vi "LVClasse_Intensity GetStatisticDatas.vi"(0 "Phase in":refnum<class "Intensity.lvclass">, 11 "error in (no error)":errorcluster) -> (4 "Phase out":refnum<class "Intensity.lvclass">, 6 "StatisticsData":T1, 15 "error out":errorcluster)   [LabVIEW 2020, in "Intensity.lvclass"]
doc: "Phase statistic data getter.\n\n--------------------------------------------------------------------------------\n\n<B>PhaseIn </B> : Phase object.\n<B>PhaseOut </B> : Phase object.\n<B>rms </B> : Phase root mean square deviation.\n<B>pv </B> : Phase peak to valley.\n<B>max </B> : Phase maximum.\n<B>min </B> : Phase minimum.\n<B>ErrorIn </B> : Error\n<B>ErrorOut </B> : Error\n\n--------------------------------------------------------------------------------"
uses:
  Intensity.lvclass
  StatisticsData.ctl
  Intensity.lvclass/Intensity.ctl
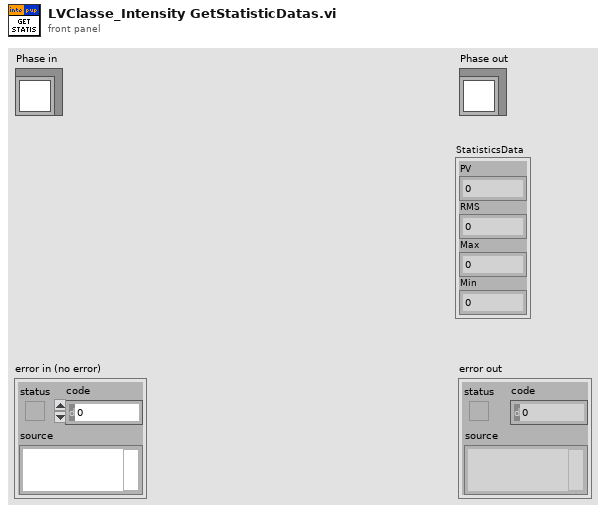
[diagram p1: front panel]
types:
  T1 = typedef "StatisticsData.ctl" = cluster{"PV":sgl, "RMS":dbl, "Max":sgl, "Min":sgl}
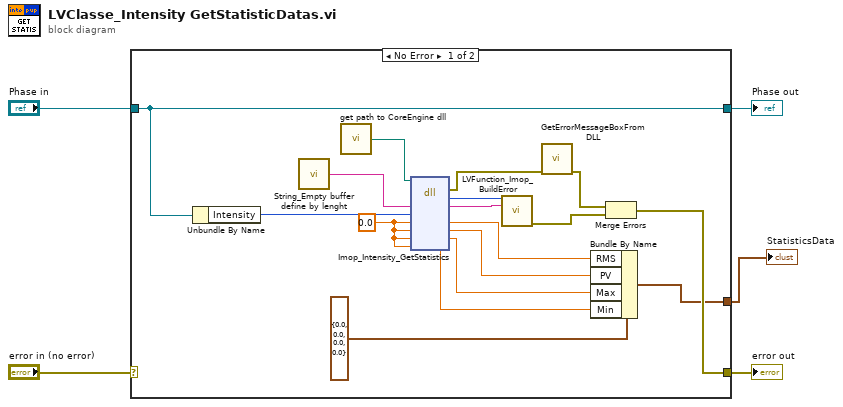
[diagram p0: block diagram]
diagram:
  n1 = case shown="No Error" "error in (no error)" {
    selector: "error in (no error)" -> [_ w24]
    tunnel: [w13 w24] -> w4
    tunnel: [w14 w23] -> w2
    tunnel: "Phase in" -> [w14 w23]
    tunnel: [w12 _] -> w1
    frame No Error {
      w6 = 0.0 ("rms")
      n2 = Unbundle By Name(w14) -> ("Intensity"=w17:i32)
      n3 = call "String_Empty buffer define by lenght.vi"() -> ("Empty buffer"=w20:string)  [unwired: 1 in]
      n4 = call "get path to CoreEngine dll.vi"() -> ("path to c_interface_vc100.dll"=w19:path)  [unwired: 12 in, 3 out]
      n5 = dll-call lib="D:/soft/HASO_v3/SVN_trunk/ImOpCoreEngine4_LV2011/DLLs/c_interface_vc100.dll" fn="Imop_Intensity_GetStatistics"(path in=w19, "message"=w20, "intensity"=w17, "rms"=w6, "PV"=w6, "max"=w6, "min"=w6) -> (error out=w18:errorcluster, "return type"=w22:i32, "message"=w21:string, "rms"=w9:dbl, "PV"=w8:dbl, "max"=w11:dbl, "min"=w10:dbl)  [unwired: 3 in, 1 out]
      n6 = call "LVFunction_Imop_BuildError.vi"("code"=w22, "String to Prepend to source (\"\")"=w21) -> ("error out"=w15:errorcluster)  [unwired: 13 in]
      n7 = call "GetErrorMessageBoxFromDLL.vi"("error IN"=w18) -> ("error OUT"=w16:errorcluster)  [unwired: 10 in]
      n8 = Bundle By Name(cluster=T1 {"PV"=0.0, "RMS"=0.0, "Max"=0.0, "Min"=0.0} ("StatisticsData"), "RMS"=w9, "PV"=w8, "Max"=w11, "Min"=w10) -> (w12:T1)
      n9 = Merge Errors(w16, w15) -> (w13:errorcluster)
    }
    frame Error {
    }
  }
  "error out" <- w4
  "Phase out" <- w2
  "StatisticsData" <- w1
